vi "Volt To Power.vi"(1 "Volt":dbl) -> (0 "Power":dbl)   [LabVIEW 2017]
uses:
  <vilib>/express/express arith-compare/Formula/XNode/ExpressFormulaBlockNode.xnode
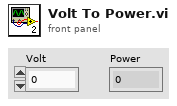
[diagram p1: front panel]
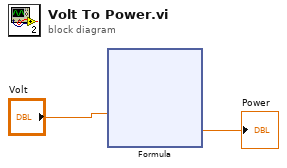
[diagram p0: block diagram]
diagram:
  n1 = xnode "Formula"("Volt"="Volt") -> ("Result"=→"Power":dbl)  [unwired: 1 in, 1 out]
